vi "CloseBlockDiagram.vi"(10 "Block Diagram":refnum<vi>, 11 "VI Reference":refnum<vi>) -> (3 "VI Name Out":string)   [LabVIEW 2012]
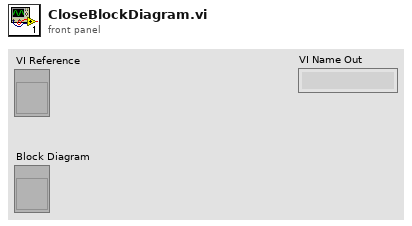
[diagram p1: front panel]
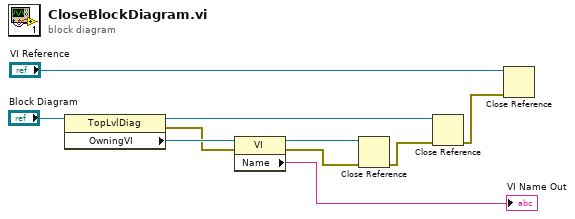
[diagram p0: block diagram]
diagram:
  n1 = property class="TopLvlDiag"(reference="Block Diagram") -> (reference out=w4:refnum<vi>, error out=w8:errorcluster, "OwningVI"=w9:refnum<vi>)  [unwired: 1 in]
  n2 = property class="VI"(reference=w9, error in=w8) -> (reference out=w6:refnum<vi>, error out=w5:errorcluster, "Name"=→"VI Name Out":string)
  n3 = Close Reference(reference=w6, error in (no error)=w5) -> (error out=w3:errorcluster)
  n4 = Close Reference(reference=w4, error in (no error)=w3) -> (error out=w1:errorcluster)
  n5 = Close Reference(reference="VI Reference", error in (no error)=w1) -> ()  [unwired: 1 out]
